vi "HEWH Convert Temp to Color.vi"(5 "Max Temp (°F)":dbl=140.0, 7 "Min Temp (°F)":dbl=50.0, 8 "Error In":errorcluster, 10 "Temp (°F)":dbl=75.0) -> (0 "Error Out":errorcluster, 2 "Control Data":T1)   [LabVIEW 2016]
uses:
  Type Definitions/HEWH Display Colors.ctl
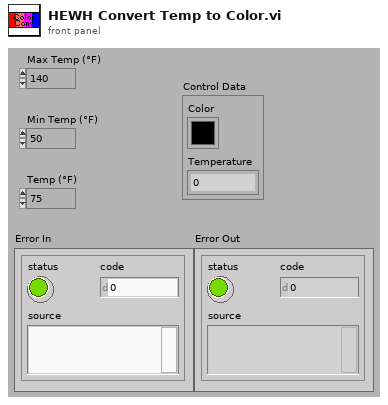
[diagram p1: front panel]
types:
  T1 = typedef "HEWH Display Colors.ctl" = cluster{"Color":u32, "Temperature":dbl}
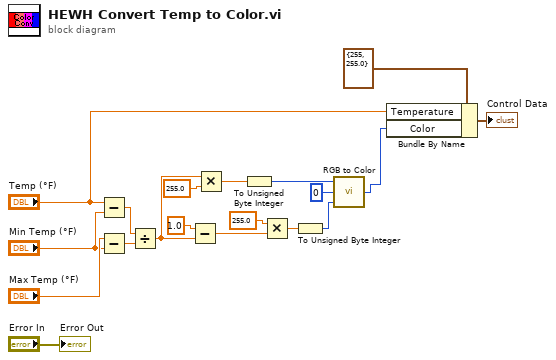
[diagram p0: block diagram]
diagram:
  n1 = Subtract(x="Temp (°F)", y="Min Temp (°F)") -> (x-y=w8:dbl)
  n2 = Subtract(x="Max Temp (°F)", y="Min Temp (°F)") -> (x-y=w9:dbl)
  n3 = Divide(x=w8, y=w9) -> (x/y=w11:dbl)
  n4 = Subtract(x=1.0, y=w11) -> (x-y=w13:dbl)
  n5 = Multiply(x=w11, y=255.0) -> (x*y=w16:dbl)
  n6 = To Unsigned Byte Integer(number=w16) -> (unsigned 8bit integer=w18:u8)
  n7 = Multiply(x=255.0 ("y"), y=w13) -> (x*y=w15:dbl)
  n8 = To Unsigned Byte Integer(number=w15) -> (unsigned 8bit integer=w19:u8)
  n9 = call <vilib>:"RGB to Color.vi"("B"=w19, "G"=u8 0, "R"=w18) -> ("Color"=w3:u32)
  n10 = Bundle By Name(cluster=T1 {"Color"=255, "Temperature"=255.0}, "Temperature"="Temp (°F)", "Color"=w3) -> (→"Control Data":T1)
  "Error Out" <- "Error In"
